vi "Get View Details.vi"(8 "error in (no error)":errorcluster, 10 "View Name":string, 11 "Controller in":refnum<class "Controller.lvclass">) -> (0 "error out":errorcluster, 2 "View Details":T1, 3 "View Found":bool)   [LabVIEW 2023, in "MVC Actors.lvlib" / "Controller.lvclass"]
uses:
  Controller.lvclass
  View Details.ctl
  <vilib>/ActorFramework/Message Enqueuer/Message Enqueuer.lvclass
  Controller.lvclass/Controller.ctl
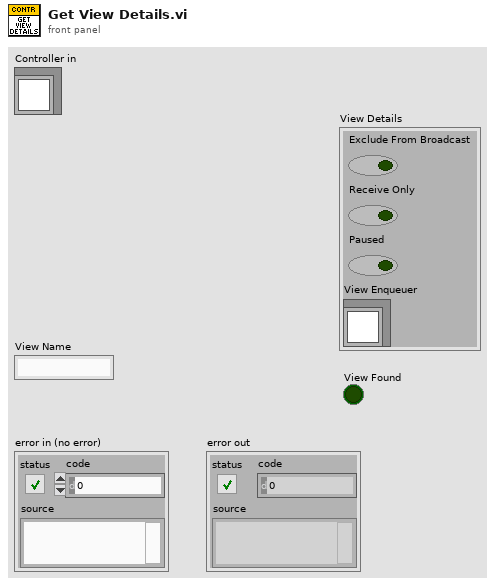
[diagram p1: front panel]
types:
  T1 = typedef "MVC Actors.lvlib/Controller.lvclass/View Details.ctl" = cluster{"Exclude From Broadcast":bool, "Receive Only":bool, "Paused":bool, "View Enqueuer":refnum<class "Message Enqueuer.lvclass">}
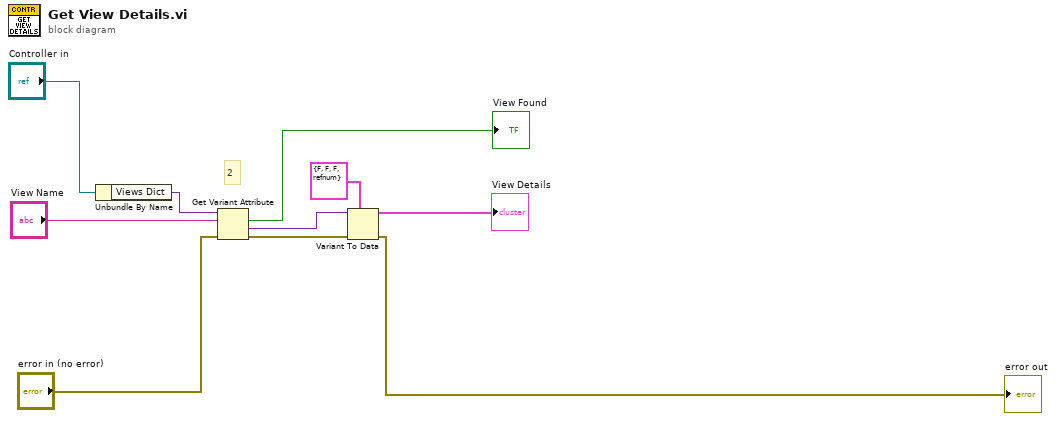
[diagram p0: block diagram]
diagram:
  # "2"
  n1 = Unbundle By Name("Controller in") -> ("Views Dict"=w8:variant)
  n2 = Get Variant Attribute(Variant=w8, name="View Name", error in="error in (no error)") -> (found=→"View Found":bool, value=w5:variant, error out=w9:errorcluster)  [unwired: 1 in, 1 out]
  n3 = Variant To Data(error in=w9, type=T1 {"Exclude From Broadcast"=FALSE, "Receive Only"=FALSE, "Paused"=FALSE, "View Enqueuer"=refnum} ("Message Enqueuer"), Variant=w5) -> (data=→"View Details":T1, error out=→"error out":errorcluster)
